vi "KillPixelsOutsideCircularROI (SubVI).vi"(1 "XY Array":dbl[][](array[numeric]), 2 "Radius*ScaleFactor":dbl, 3 "Center (Pixels)":cluster{"X":sgl, "Y":sgl}) -> (0 "subarray":dbl[][](array[numeric]))   [LabVIEW 2016]
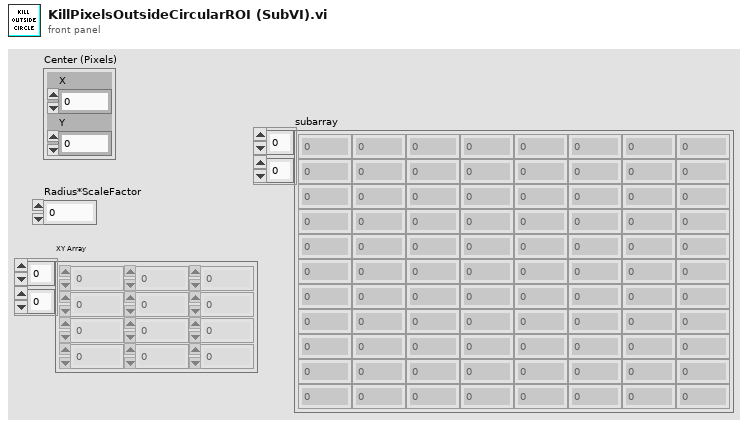
[diagram p1: front panel]
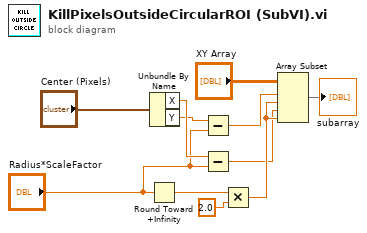
[diagram p0: block diagram]
diagram:
  n1 = Round Toward +Infinity(x="Radius*ScaleFactor") -> (ceil(x): smallest int >= x=w7:dbl)
  n2 = Unbundle By Name("Center (Pixels)") -> ("X"=w10:sgl, "Y"=w9:sgl)
  n3 = Subtract(x=w9, y="Radius*ScaleFactor") -> (x-y=w1:dbl)
  n4 = Subtract(x=w10, y="Radius*ScaleFactor") -> (x-y=w2:dbl)
  n5 = Multiply(x=w7, y=2.0) -> (x*y=w5:dbl)
  n6 = Array Subset(array="XY Array", index (row)=w1, length (row)=w5, index (col)=w2, length (col)=w5) -> (→"subarray":dbl[][])
